vi "NetClient.vi"(1 "Port":u16) -> ()   [LabVIEW 2013]
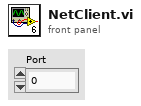
[diagram p1: front panel]
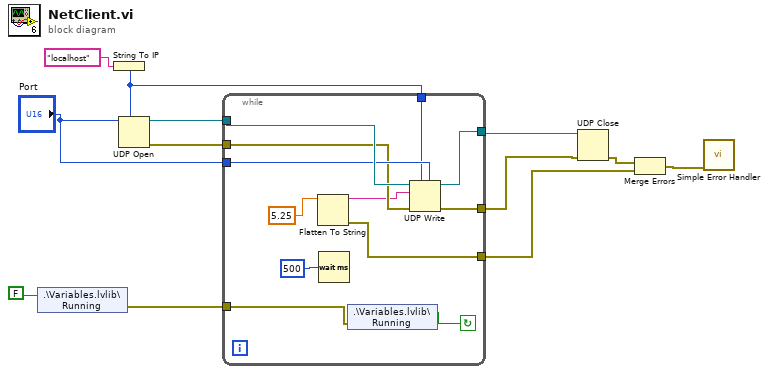
[diagram p0: block diagram]
diagram:
  n1 = shared-variable ".\\Variables.lvlib\\Running"(FALSE) -> (error out=w8:errorcluster)  [unwired: 1 in]
  n2 = String To IP(1:"localhost") -> (0:w1:u32)
  n3 = UDP Open(7:w1, 11:"Port") -> (port=w11:refnum<k16>, 0:w6:errorcluster)  [unwired: 3 in, 1 out]
  n4 = while {
    tunnel: w11 -> [w23]
    tunnel: [w22] -> w10
    tunnel: "Port" -> [w21]
    tunnel: w1 -> [w20]
    tunnel: w8 -> [w19]
    tunnel: w6 -> [w18]
    tunnel: [w17] -> w5
    tunnel: [w16] -> w3
    stop <- w24 continue-if-true
    n5 = Flatten To String(anything=5.25) -> (data string=w13:string, error out=w17:errorcluster)  [unwired: 3 in, 1 out]
    n6 = Wait (ms)(milliseconds to wait=500) -> ()  [unwired: 1 out]
    n7 = shared-variable ".\\Variables.lvlib\\Running"(error in=w19) -> (w24:bool)  [unwired: 1 out]
    n8 = UDP Write(address=w20, port or service name=w21, connection ID=w23, data in=w13, 8:w18) -> (error out=w16:errorcluster, 3:w22:refnum<k16>)  [unwired: 1 in]
  }
  n9 = UDP Close(connection ID=w10, 8:w3) -> (error out=w7:errorcluster)  [unwired: 1 out]
  n10 = Merge Errors(w7, w5) -> (w4:errorcluster)
  n11 = call <vilib>:"Simple Error Handler.vi"("error in (no error)"=w4) -> ()  [unwired: 4 in, 5 out]
